vi "Update-Velocity.vi"(8 "Error In":errorcluster) -> (0 "Error Out":errorcluster, 3 "Velocity":dbl)   [LabVIEW 2017]
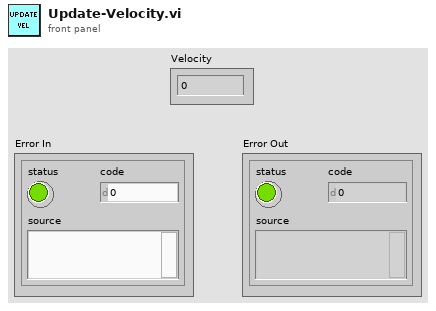
[diagram p1: front panel]
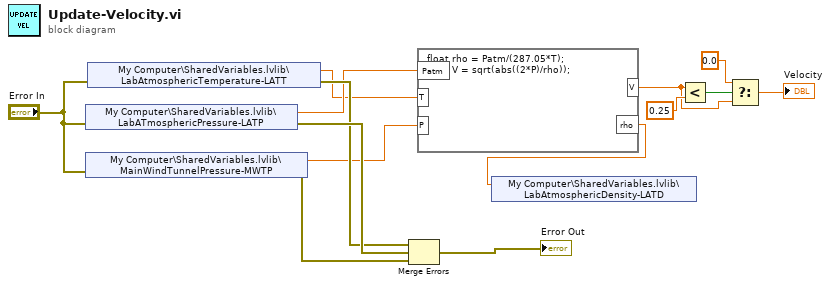
[diagram p0: block diagram]
diagram:
  n1 = shared-variable "My Computer\\SharedVariables.lvlib\\LabATmosphericPressure-LATP"(error in="Error In") -> (w11:dbl, error out=w14:errorcluster)
  n2 = shared-variable "My Computer\\SharedVariables.lvlib\\MainWindTunnelPressure-MWTP"(error in="Error In") -> (w7:dbl, error out=w8:errorcluster)
  n3 = shared-variable "My Computer\\SharedVariables.lvlib\\LabAtmosphericTemperature-LATT"(error in="Error In") -> (w10:dbl, error out=w13:errorcluster)
  n4 = Merge Errors(w13, w14, w8) -> (→"Error Out":errorcluster)
  n5 = formula code="float rho = Patm/(287.05*T);\nfloat V = sqrt(abs((2*P)/rho));"("Patm"=w11, "T"=w10, "P"=w7) -> ("V"=w2:dbl, "rho"=w6:dbl)
  n6 = shared-variable "My Computer\\SharedVariables.lvlib\\LabAtmosphericDensity-LATD"(w6) -> ()  [unwired: 1 in, 1 out]
  n7 = Less?(x=w2, y=0.25) -> (x < y?=w4:bool)
  n8 = Select(t=0.0, s=w4, f=w2) -> (s? t:f=→"Velocity":dbl)
